vi "Encoder Get.vi"(9 "Use in Simulator (F)":bool, 11 "refnum name":string="My Encoder RefNum") -> (1 "Distance":dbl)   [LabVIEW 2012]
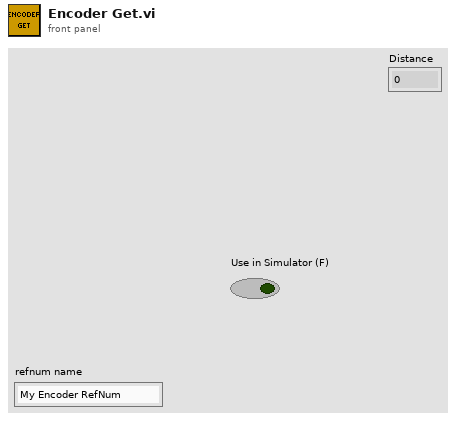
[diagram p1: front panel]
types:
  T1 = typedef "WPI_EncoderDevRef.ctl" = cluster{"DevStatus":errorcluster, "EncoderIndex":T2, "CounterIndex":T3, "DistancePerCount":dbl, "Decoding Type":T4}
  T2 = typedef "FPGA_EncoderIdx.ctl" = enum8{"Enc 0", "Enc 1", "Enc 2", "Enc 3", "Invalid"}
  T3 = typedef "FPGA_CounterCtrSystemIndex.ctl" = enum8{"Ctr 0", "Ctr 1", "Ctr 2", "Ctr 3", "Ctr 4", "Ctr 5", "Ctr 6", "Ctr 7", "Invalid"}
  T4 = typedef "WPI_EncoderType.ctl" = enum16{"1x", "2x", "4x"}
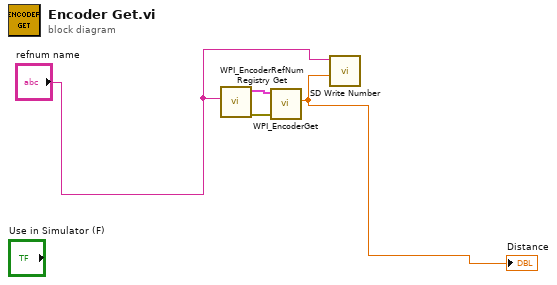
[diagram p0: block diagram]
diagram:
  n1 = call <vilib>:"WPI_EncoderRefNum Registry Get.vi"("refnum name"="refnum name") -> ("error out"=w1:errorcluster, "EncoderDevRef"=w4:T1)  [unwired: 9 in]
  n2 = call <vilib>:"WPI_EncoderGet.vi"("error in (no error)"=w1, "EncoderDevRef"=w4) -> ("Distance"=w2:dbl)  [unwired: 4 in, 5 out]
  "Distance" <- w2
  n3 = call <vilib>:"SD Write Number.vi"("Numeric"=w2, "Name"="refnum name") -> ()  [unwired: 8 in, 2 out]
